vi "waveDblTest.vi"() -> ()   [LabVIEW 2018]
panel:
  out "result string":string="\\documentclass[convert={density=400,outext=.png}]{standalone}\n\\usepackage[utf8]{inputenc}\n\\usepackage{pgfplots}\n\\pgfplotsset{width=15cm,compat=newest}\n\n\n\\begin{document}\n\n\\begin{tikzpicture}\n\\begin{axis}[xmin=0.000000, xmax=5.000000, ymin=-3.000000, ymax=4.000000, xlabel=Time, ylabel=Amplitude]\n\n\\definecolor{myColor0}{RGB}{200, 174, 0}\n\\addplot[color=myColor0, mark= , solid] coordinates { (0.000000,1.000000) (1.000000,1.000000) (2.000000,2.000000) (3.000000,2.000000) (4.000000,3.000000) (5.000000,2.000000)};\n\\addlegendentry{Plot 0}\n\\definecolor{myColor1}{RGB}{255, 66, 66}\n\\addplot[color=myColor1, mark= , solid] coordinates { (0.000000,2.000000) (1.000000,-2.000000) (2.000000,0.000000) (3.000000,4.000000) (4.000000,-3.000000) (5.000000,4.000000)};\n\\addlegendentry{Plot 1}\n\\definecolor{myColor2}{RGB}{14, 255, 0}\n\\addplot[color=myColor2, mark= , solid] coordinates { (0.000000,-2.000000) (1.000000,-2.000000) (2.000000,2.000000) (3.000000,2.000000) (4.000000,2.000000) (5.000000,2.000000)};\n\\addlegendentry{Plot 2}\n\\end{axis}\n\\end{tikzpicture}\n\n\\end{document}"
  out "Waveform Graph":dbl[][](graph)=[[1.0, 1.0, 2.0, 2.0, 3.0, 2.0], [2.0, -2.0, 0.0, 4.0, -3.0, 4.0], [-2.0, -2.0, 2.0, 2.0, 2.0, 2.0]]
  in  "Array 3":dbl[](array[numeric])=[-2.0, -2.0, 2.0, 2.0, 2.0, 2.0]
  in  "Array 2":dbl[](array[numeric])=[2.0, -2.0, 0.0, 4.0, -3.0, 4.0]
  in  "Array":dbl[](array[numeric])=[1.0, 1.0, 2.0, 2.0, 3.0, 2.0]
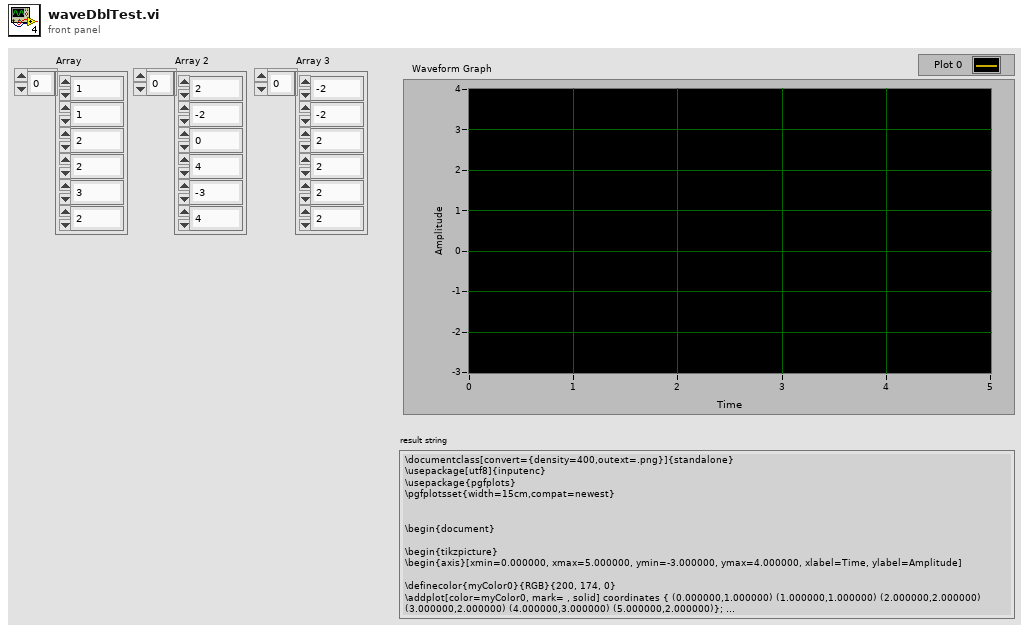
[diagram p1: front panel]
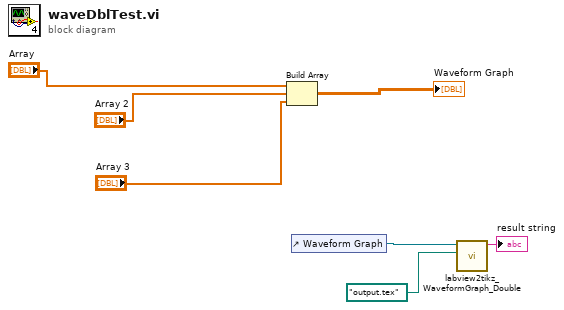
[diagram p0: block diagram]
diagram:
  n1 = Build Array("Array", "Array 2", "Array 3") -> (→"Waveform Graph":dbl[][])
  n2 = control-ref of="Waveform Graph"() -> (w3:refnum<vi>)
  n3 = call "labview2tikz_WaveformGraph_Double.vi"("file (use dialog)"=path "output.tex", "Waveform Graph"=w3) -> ("result string"=→"result string":string)  [unwired: 8 in, 1 out]
